vi "XCP Log Parser.vi"(5 "DTO IDs":u32[](array[numeric]) caption="Specify your own DTO_IDs" format="%.0x", 7 "Get DIO_ID from A2L":bool=TRUE, 8 "Output Directory":path=path "C:/LVLibrary/XNET/XCP_DaqDtoID/XCP_DaqDtoId", 9 "Generate Database":bool=TRUE, 10 "XCP Log File":path=path "C:/LVLibrary/XNET/XCP_DaqDtoID/XCP_DaqDtoId/ECUMCLog/XCP_MeasSplit.xlg", 11 "A2L File Path":path=path "C:/LVLibrary/XNET/XCP_DaqDtoID/s3_svn11341.a2l") -> (0 "Error Out":errorcluster, 2 "Measurement Signals":refnum<k21>[](array[refnum]), 3 "DAQList out":refnum<class "DAQList.lvclass">)   [LabVIEW 2019, in "XCP_DaqDtoId.lvlib" / "DAQList.lvclass"]
uses:
  DAQList.lvclass
  TypeDef/SpecialFlag.ctl
  <vilib>/ECUMC/ECUMC.llb/MC Get Names Type.ctt
  DAQList.lvclass/DAQList.ctl
  A2L_Utility/Private/Find CAN_ID.vi
  DatabaseGeneration/SubVI_SetMeasProp.vi
  DatabaseGeneration/SubVI_ProcessMeasName.vi
  A2L_Utility/Private/ParseNumeric.vi
  <vilib>/ECUMC/ECUMC.llb/MC Get Property.vi
  <vilib>/ECUMC/ECUMC.llb/MC Get Prop DB File Name.vi
  <vilib>/Utility/file.llb/Read Delimited Spreadsheet.vi
  <vilib>/Utility/file.llb/Read Delimited Spreadsheet (string).vi
  <vilib>/Utility/error.llb/Error Cluster From Error Code.vi
  <vilib>/ECUMC/ECUMC.llb/MC Get Prop XCP DTO Id.vi
  <vilib>/ECUMC/ECUMC.llb/MC Get Prop XCP CRO Id.vi
  <vilib>/ECUMC/ECUMC.llb/MC Get Prop XCP CAN IO Mode.vi
  <vilib>/ECUMC/ECUMC.llb/MC Get Prop XCP Baud Rate 64.vi
  <vilib>/ECUMC/ECUMC.llb/MC Get Prop XCP FD Baud Rate 64.vi
  <vilib>/xnet/xnet.llb/XNET Database Create Object.vi
  <vilib>/xnet/xnet.llb/XNET Database Create (Cluster).vi
  <vilib>/xnet/xnet.llb/XNET Database Create (Frame).vi
  <vilib>/Utility/file.llb/Application Directory.vi
  <vilib>/xnet/xnet.llb/XNET Database Save.vi
  <vilib>/ECUMC/ECUMC.llb/MC Get Prop Meas Address.vi
  <vilib>/xnet/xnet.llb/XNET Database Create (Signal).vi
  <vilib>/xnet/xnet.llb/XNET Database Create (Subframe).vi
  <vilib>/ECUMC/ECUMC.llb/MC Get Prop Meas Data Type.vi
  TypeDef/Global.vi
  <vilib>/xnet/xnet.llb/XNET Database Create (Dynamic Signal).vi
  <vilib>/ECUMC/ECUMC.llb/MC Get Prop Meas Comment.vi
  <vilib>/ECUMC/ECUMC.llb/MC Get Prop Meas Scaling Offset.vi
  <vilib>/ECUMC/ECUMC.llb/MC Get Prop Meas Scaling Factor.vi
  <vilib>/ECUMC/ECUMC.llb/MC Get Prop Meas Minimum.vi
  <vilib>/ECUMC/ECUMC.llb/MC Get Prop Meas Maximum.vi
  <vilib>/ECUMC/ECUMC.llb/MC Get Prop Meas Byte Order.vi
  <vilib>/ECUMC/ECUMC.llb/MC Get Prop Meas Unit.vi
  <vilib>/ECUMC/ECUMC.lvlib
  A2L Utility.lvlib
panel:
  in  "Special Flag":T1
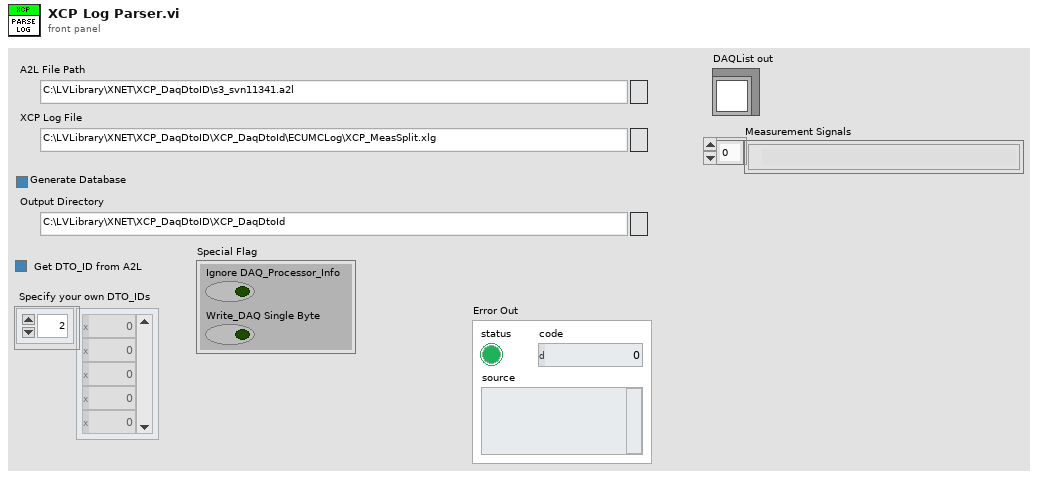
[diagram p1: front panel]
types:
  T1 = typedef "XCP_DaqDtoId.lvlib/DAQList.lvclass/SpecialFlag.ctl" = cluster{"Ignore DAQ_Processor_Info":bool, "Write_DAQ Single Byte":bool}
  T2 = typedef "ECUMC.lvlib/MC Get Names Type.ctt" = u32
  T3 = typedef "ECUMC.lvlib/MC Reference.ctt" = u32
  T4 = typedef "XNET Frame CAN.ctl" = cluster{"timestamp":timestamp, "payload":u8[], "identifier":u32, "type":T5, "extended?":bool, "echo?":bool}
  T5 = typedef "XNET Frame Type CAN.ctl" = u8
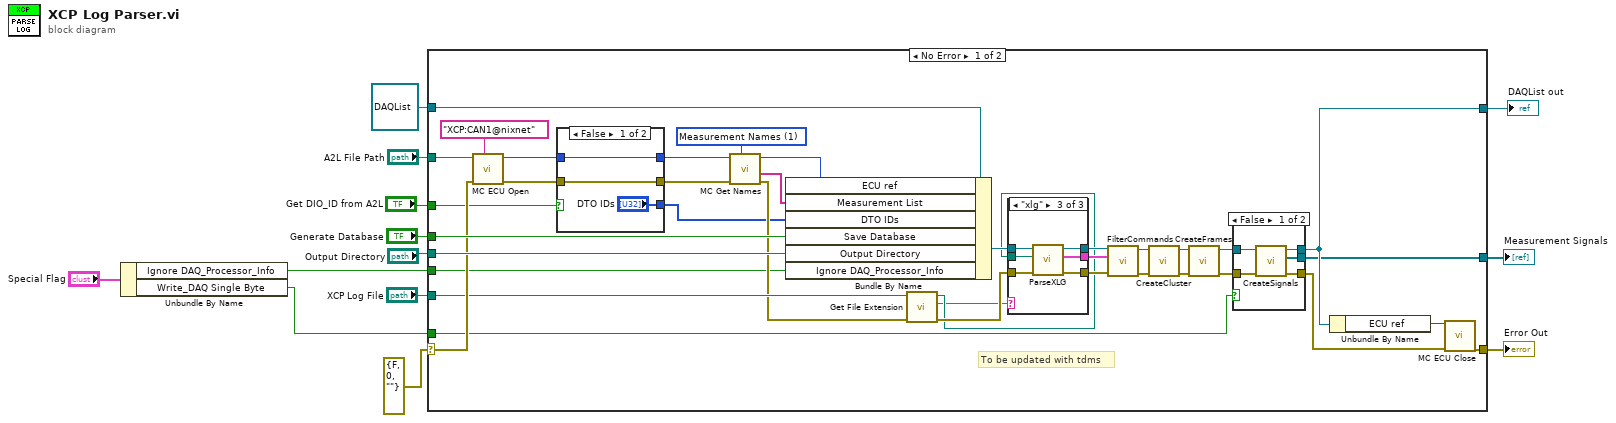
[diagram p0: block diagram]
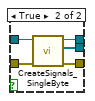
[diagram p2: hidden frame]
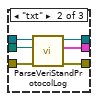
[diagram p4: hidden frame]
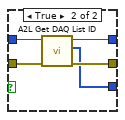
[diagram p5: hidden frame]
diagram:
  n1 = Unbundle By Name("Special Flag") -> ("Ignore DAQ_Processor_Info"=w2:bool, "Write_DAQ Single Byte"=w1:bool)
  n2 = case shown="No Error" errorcluster {"status"=FALSE, "code"=0, "source"=""} ("error IO") {
    selector: errorcluster {"status"=FALSE, "code"=0, "source"=""} ("error IO") -> [w45 w84]
    tunnel: [w35 w84] -> w7
    tunnel: [w17 w83] -> w13
    tunnel: refnum<class "DAQList.lvclass"> refnum ("DAQList out") -> [w50 w83]
    tunnel: "Output Directory" -> [w49 _]
    tunnel: "Generate Database" -> [w48 _]
    tunnel: "A2L File Path" -> [w47 _]
    tunnel: "XCP Log File" -> [w40 _]
    tunnel: "Get DIO_ID from A2L" -> [w20 _]
    tunnel: [w16 _] -> w4
    tunnel: w2 -> [w15 _]
    tunnel: w1 -> [w14 _]
    frame No Error {
      w26 = T2 1 items=["ECU Names", "Measurement Names", "Characteristic Names", "Event Channel Names", "Defined Pages Names", "Group Names", "Group - Subgroup Names", "Group - Measurement Names", "Group - Characteristic Names", "Function Names", "Function - DefCharacteristic Names", "Function - RefCharacteristic Names", "Function - InMeasurement Names", "Function - OutMeasurement Names", "Function - LocMeasurement Names", "Function - SubFunction Names", "Group - Function List Names", "XCP on CAN - Transport Layer Instance Names", "XCP on TCP - Transport Layer Instance Names", "XCP on UDP - Transport Layer Instance Names"] ("type")
      # "To be updated with tdms"
      n3 = call <vilib>:"MC ECU Open.vi"("protocol and interface"="XCP:CAN1@nixnet", "error in"=w45, "DB path"=w47) -> ("error out"=w27:errorcluster, "ECU ref out"=w28:T3)  [unwired: 7 in]
      n4 = case shown="False" w20 {
        tunnel: w28 -> [w77 w82]
        tunnel: w27 -> [w76 w81]
        tunnel: [w77 w80] -> w25
        tunnel: [w76 w79] -> w22
        tunnel: ["DTO IDs" w78] -> w19
        frame False {
        }
        frame True {
          n5 = call "A2L Get DAQ List ID.vi"("error in (no error)"=w81, "ECU ref in"=w82) -> ("error out"=w79:errorcluster, "DAQ List IDs"=w78:u32[], "ECU ref out"=w80:T3)  [unwired: 7 in]
        }
      }
      n6 = call <vilib>:"MC Get Names.vi"("type"=w26, "error in"=w22, "reference in"=w25) -> ("error out"=w21:errorcluster, "names list out"=w24:string[], "reference out"=w23:T3)  [unwired: 1 in, 5 out]
      n7 = Bundle By Name(cluster=w50, "ECU ref"=w23, "Measurement List"=w24, "DTO IDs"=w19, "Save Database"=w48, "Output Directory"=w49, "Ignore DAQ_Processor_Info"=w15) -> (w43:refnum<class "DAQList.lvclass">)
      n8 = call <vilib>:"Get File Extension.vi"("error in (no error)"=w21, "file"=w40) -> ("error out"=w39:errorcluster, "lowercase file extension"=w37:string, "dup file"=w38:path)  [unwired: 5 in, 2 out]
      n9 = case shown="\"xlg\"" w37 {
        tunnel: [w62 w68 w71] -> w44
        tunnel: w43 -> [w62 w67 w74]
        tunnel: w39 -> [w61 w66 w72]
        tunnel: [w61 w65 w69] -> w42
        tunnel: [_ w64 w70] -> w41
        tunnel: w38 -> [_ w63 w73]
        frame Default {
        }
        frame "txt" {
          n10 = call "ParseVeriStandProtocolLog.vi"("error in (no error)"=w66, "Path"=w63, "DAQList in"=w67) -> ("error out"=w65:errorcluster, "CAN Frames"=w64:T4[], "DAQList out"=w68:refnum<class "DAQList.lvclass">)  [unwired: 6 in]
        }
        frame "xlg" {
          n11 = call "ParseXLG.vi"("error in (no error)"=w72, "Path"=w73, "DAQList in"=w74) -> ("error out"=w69:errorcluster, "CAN Frames"=w70:T4[], "DAQList out"=w71:refnum<class "DAQList.lvclass">)  [unwired: 6 in]
        }
      }
      n12 = call "FilterCommands.vi"("error in (no error)"=w42, "CAN Frames"=w41, "DAQList in"=w44) -> ("error out"=w33:errorcluster, "DAQList out"=w34:refnum<class "DAQList.lvclass">)  [unwired: 7 in]
      n13 = call "CreateCluster.vi"("error in (no error)"=w33, "DAQList in"=w34) -> ("error out"=w31:errorcluster, "DAQList out"=w32:refnum<class "DAQList.lvclass">)  [unwired: 8 in]
      n14 = call "CreateFrames.vi"("error in (no error)"=w31, "DAQList in"=w32) -> ("error out"=w29:errorcluster, "DAQList out"=w30:refnum<class "DAQList.lvclass">)  [unwired: 8 in]
      n15 = case shown="False" w14 {
        tunnel: w30 -> [w55 w60]
        tunnel: w29 -> [w54 w56]
        tunnel: [w53 w57] -> w18
        tunnel: [w52 w59] -> w17
        tunnel: [w51 w58] -> w16
        frame False {
          n16 = call "CreateSignals.vi"("error in (no error)"=w54, "DAQList in"=w55) -> ("error out"=w53:errorcluster, "Measurement Signals"=w51:refnum<k21>[], "DAQList out"=w52:refnum<class "DAQList.lvclass">)  [unwired: 7 in]
        }
        frame True {
          n17 = call "CreateSignals_SingleByte.vi"("error in (no error)"=w56, "DAQList in"=w60) -> ("error out"=w57:errorcluster, "Measurement Signals"=w58:refnum<k21>[], "DAQList out"=w59:refnum<class "DAQList.lvclass">)  [unwired: 7 in]
        }
      }
      n18 = Unbundle By Name(w17) -> ("ECU ref"=w36:T3)
      n19 = call <vilib>:"MC ECU Close.vi"("error in"=w18, "ECU ref in"=w36) -> ("error out"=w35:errorcluster)  [unwired: 9 in]
    }
    frame Error {
    }
  }
  "DAQList out" <- w13
  "Error Out" <- w7
  "Measurement Signals" <- w4
